vi "Get Installed SR Type.vi"(8 "error in (no error)":errorcluster, 11 "VISA Refnum in":refnum<visa-resource-name>="COM1") -> (0 "error out":errorcluster, 2 "SR":string, 3 "VISA Refnum out":refnum<visa-resource-name>)   [LabVIEW 2019, in "KH7008.lvlib"]
uses:
  KH7008.lvlib
  typedefs/shunt--enum.ctl
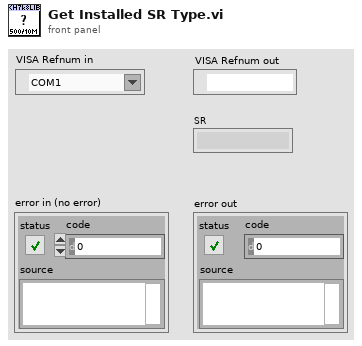
[diagram p1: front panel]
types:
  T1 = typedef "KH7008.lvlib/shunt--enum.ctl" = enum16{"Open", "50", "500", "5k", "50k", "10M"}
  T2 = typedef "KH7008.lvlib/allChannelProperties--Array.ctl" = T3[]
  T3 = typedef "KH7008.lvlib/channelProperties--Cluster.ctl" = cluster{"channel":T4, "gain":T5, "input":T6, "shunt":T1, "couple":T7, "filter":T8}
  T4 = typedef "KH7008.lvlib/channel--enum.ctl" = enum16{"1", "2", "3", "4", "5", "6", "7", "8"}
  T5 = typedef "KH7008.lvlib/gain--enum.ctl" = enum16{"1x", "10x", "100x", "1000x"}
  T6 = typedef "KH7008.lvlib/input--enum.ctl" = enum16{"OFF", "SE+", "SE-", "DIFF"}
  T7 = typedef "KH7008.lvlib/couple--enum.ctl" = enum16{"AC", "DC"}
  T8 = typedef "KH7008.lvlib/filter--enum.ctl" = enum16{"OFF", "ON"}
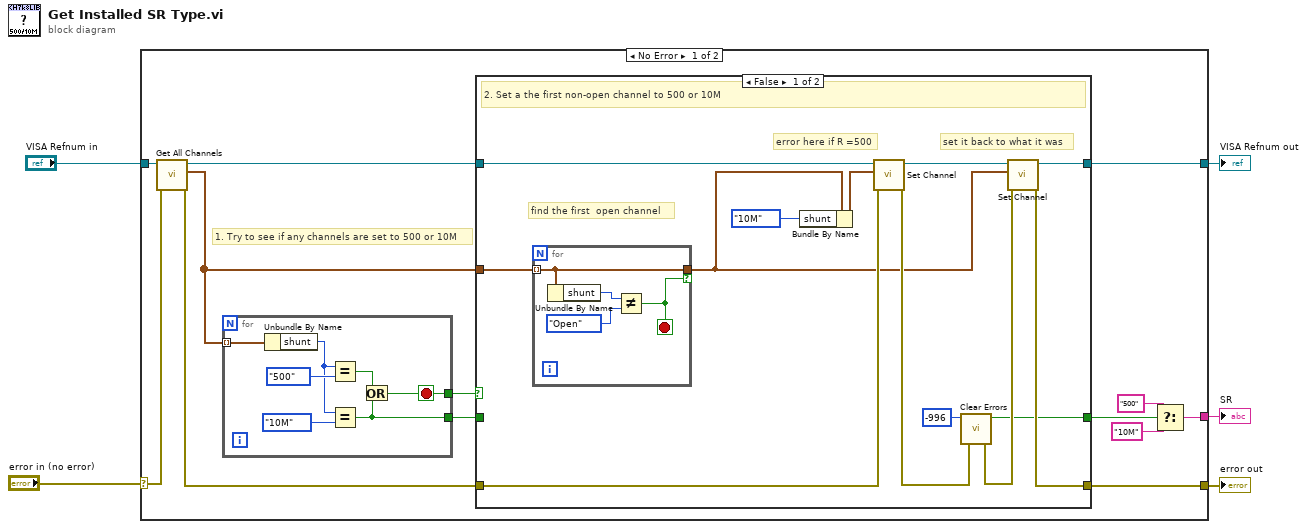
[diagram p0: block diagram]
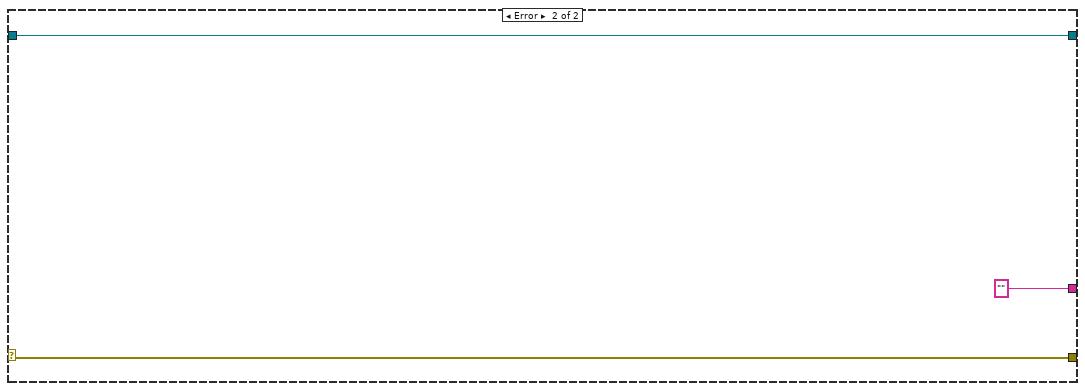
[diagram p3: hidden frame]
diagram:
  n1 = case shown="No Error" "error in (no error)" {
    selector: "error in (no error)" -> [w17 w46]
    tunnel: "VISA Refnum in" -> [w18 w48]
    tunnel: [w10 w48] -> w3
    tunnel: [w9 ""] -> w2
    tunnel: [w8 w46] -> w1
    frame No Error {
      # "1. Try to see if any channels are set to 500 or 10M"
      n2 = call "Get All Channels.vi"("error in (no error)"=w17, "VISA Refnum in"=w18) -> ("error out"=w16:errorcluster, "Channel Parameters out"=w13:T2, "VISA Refnum out"=w14:refnum<visa-resource-name>)  [unwired: 7 in]
      n3 = for {
        tunnel: w13 -> [w25] mode=indexing
        tunnel: [w20] -> w15
        tunnel: [w19] -> w12
        stop <- w20 stop-if-true
        n4 = Unbundle By Name(w25) -> ("shunt"=w22:T1)
        n5 = Equal?(x=w22, y=shunt--enum."500" ("shunt")) -> (x = y?=w21:bool)
        n6 = Equal?(x=w22, y=shunt--enum."10M" ("shunt")) -> (x = y?=w19:bool)
        n7 = Or(x=w21, y=w19) -> (x .or. y?=w20:bool)
      }
      n8 = case shown="False" w15 {
        tunnel: w16 -> [w35 w43]
        tunnel: w14 -> [w37 w44]
        tunnel: w13 -> [w38 _]
        tunnel: w12 -> [_ w45]
        tunnel: [w27 w45] -> w11
        tunnel: [w30 w44] -> w10
        tunnel: [w29 w43] -> w8
        frame False {
          # "find the first  open channel"
          # "set it back to what it was"
          # "error here if R =500"
          # "2. Set a the first non-open channel to 500 or 10M"
          n9 = for {
            tunnel: w38 -> [w40] mode=indexing
            tunnel: [w40] -> w28 if=w39
            stop <- w39 stop-if-true
            n10 = Unbundle By Name(w40) -> ("shunt"=w42:T1)
            n11 = Not Equal?(x=w42, y=shunt--enum."Open" ("shunt")) -> (x != y?=w39:bool)
          }
          n12 = Bundle By Name(cluster=w28, "shunt"=shunt--enum."10M") -> (w36:T3)
          n13 = call "Set Channel.vi"("error in (no error)"=w35, "channelParameter"=w36, "VISA Refnum in"=w37) -> ("error out"=w32:errorcluster, "VISA Refnum out"=w33:refnum<visa-resource-name>)  [unwired: 7 in]
          n14 = call <vilib>:"Clear Errors.vi"("error in (no error)"=w32, "specific error code to clear (0: all)"=-996) -> ("error out"=w31:errorcluster, "specific error cleared?"=w27:bool)  [unwired: 4 in]
          n15 = call "Set Channel.vi"("error in (no error)"=w31, "channelParameter"=w28, "VISA Refnum in"=w33) -> ("error out"=w29:errorcluster, "VISA Refnum out"=w30:refnum<visa-resource-name>)  [unwired: 7 in]
        }
        frame True {
          # "1.One of the channels was 500 or 10M"
        }
      }
      n16 = Select(t="500", s=w11, f="10M") -> (s? t:f=w9:string)
    }
    frame Error {
    }
  }
  "VISA Refnum out" <- w3
  "error out" <- w1
  "SR" <- w2
